vi "Chanel Names.vi"(7 "Write?":bool, 8 "error in":errorcluster, 10 "Channel Names":T1={"A-1,  1"="Main", "A-3,  2"="Main", "A-4, 3"="Recirculation", "A-5, 4"="Scrubber", "ABCD-7, 5"="Oxygen", "D-8, 6"="Vent", "B-1,  7"="Boost A", "B-3, 8"="Boost A", "B-4,  9"="Recirculation", "B-5, 10"="Scrubber", "B-8, 11"="Vent", "C-1, 12"="Boost B", "C-3, 13"="Boost B", "C-4, 14"="Recirculation", "C-5,  15"="Scrubber", "C-8, 16"="Vent", "D-1, 17"="+24V", "D-3, 18"="Main", "D-4,  19"="Boost A", "D-5,  20"="Boost B", "D-8,  21"="Vent"}, 11 "CfgFileIn":T2) -> (0 "error out":errorcluster, 2 "Channel Names Out":T1={"A-1,  1"="Main", "A-3,  2"="Main", "A-4, 3"="Recirculation", "A-5, 4"="Scrubber", "ABCD-7, 5"="Oxygen", "D-8, 6"="Vent", "B-1,  7"="Boost A", "B-3, 8"="Boost A", "B-4,  9"="Recirculation", "B-5, 10"="Scrubber", "B-8, 11"="Vent", "C-1, 12"="Boost B", "C-3, 13"="Boost B", "C-4, 14"="Recirculation", "C-5,  15"="Scrubber", "C-8, 16"="Vent", "D-1, 17"="+24V", "D-3, 18"="Main", "D-4,  19"="Boost A", "D-5,  20"="Boost B", "D-8,  21"="Vent"}, 3 "CfgFileOut":T2)   [LabVIEW 2012]
uses:
  <vilib>/Utility/config.llb/Config Data RefNum.ctl
  Type Defs/Named Final Output name list ordered.ctl
  <vilib>/Utility/config.llb/Write Key (String).vi
  <vilib>/Utility/config.llb/Read Key (String).vi
  <vilib>/Utility/config.llb/NI_LVConfig.lvlib
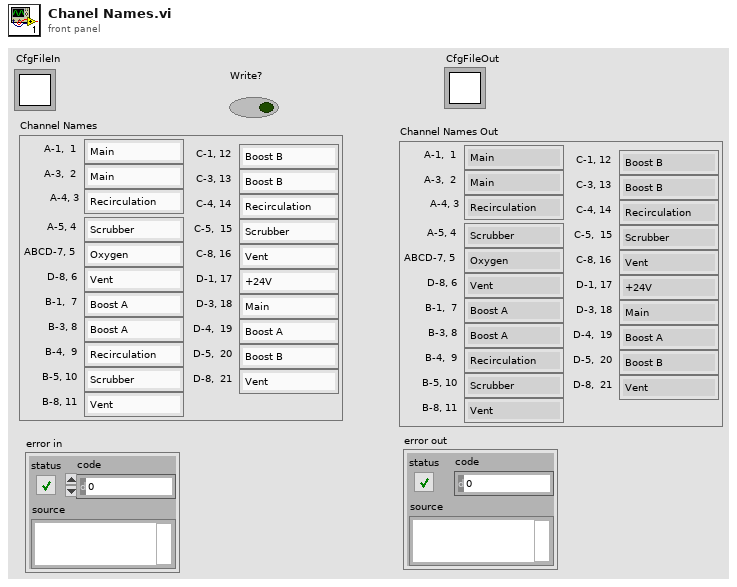
[diagram p1: front panel]
types:
  T1 = typedef "Named Final Output name list ordered.ctl" = cluster{"A-1,  1":string, "A-3,  2":string, "A-4, 3":string, "A-5, 4":string, "ABCD-7, 5":string, "D-8, 6":string, "B-1,  7":string, "B-3, 8":string, "B-4,  9":string, "B-5, 10":string, "B-8, 11":string, "C-1, 12":string, "C-3, 13":string, "C-4, 14":string, "C-5,  15":string, "C-8, 16":string, "D-1, 17":string, "D-3, 18":string, "D-4,  19":string, "D-5,  20":string, "D-8,  21":string}
  T2 = typedef "NI_LVConfig.lvlib/Config Data RefNum.ctl" = refnum<k1>
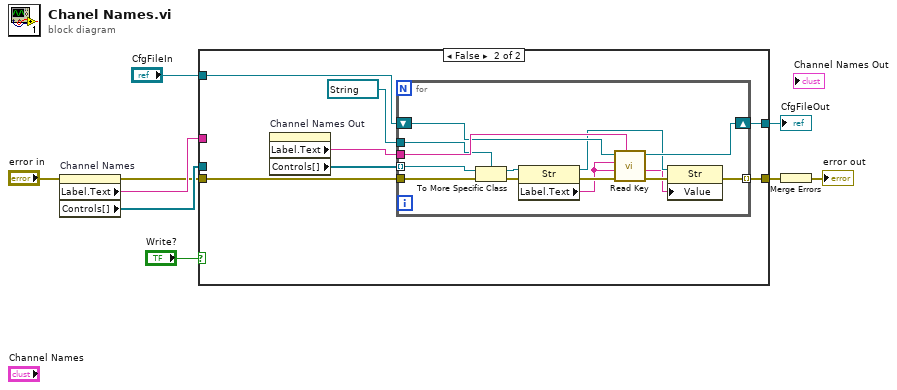
[diagram p0: block diagram]
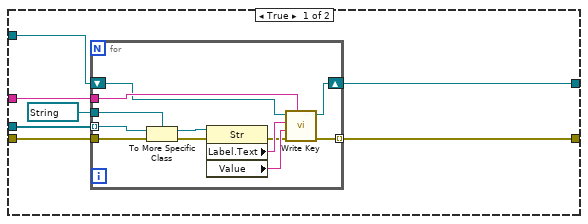
[diagram p2: hidden frame]
diagram:
  n1 = property on="Channel Names" class="Clust (strict)"(error in="error in") -> (error out=w4:errorcluster, "Label.Text"=w8:string, "Controls[]"=w9:refnum<vi>[])  [unwired: 1 in, 1 out]
  n2 = case shown="False" "Write?" {
    tunnel: w9 -> [w16 _]
    tunnel: w8 -> [w15 _]
    tunnel: "CfgFileIn" -> [w13 w34]
    tunnel: [w12 w33] -> w6
    tunnel: w4 -> [w11 w32]
    tunnel: [w10 w31] -> w3
    frame True {
      n3 = for {
        tunnel: w16 -> [w27] mode=indexing
        tunnel: w15 -> [w28]
        tunnel: refnum<vi> refnum ("Str Refnum") -> [w26]
        shift-right: [w20] -> w12
        shift-left: w13 -> [w23]
        tunnel: w11 -> [w19]
        tunnel: [w17] -> w10 mode=indexing
        n4 = To More Specific Class(target class=w26, reference=w27, error in=w19) -> (specific class reference=w25:refnum<vi>, error out=w24:errorcluster)
        n5 = property class="Str"(reference=w25, error in=w24) -> (error out=w18:errorcluster, "Label.Text"=w22:string, "Value"=w21:string)  [unwired: 1 out]
        n6 = call-poly <vilib>:"Write Key.vi"("section"=w28, "error in (no error)"=w18, "value"=w21, "key"=w22, "refnum"=w23) -> ("error out"=w17:errorcluster, "refnum out"=w20:T2)  [unwired: 4 in, 1 out]
      }
    }
    frame False {
      n7 = property on="Channel Names Out" class="Clust (strict)"() -> ("Label.Text"=w30:string, "Controls[]"=w29:refnum<vi>[])  [unwired: 2 in, 2 out]
      n8 = for {
        tunnel: w29 -> [w40] mode=indexing
        tunnel: w30 -> [w49]
        tunnel: refnum<vi> refnum ("Str Refnum") -> [w48]
        shift-right: [w44] -> w33
        shift-left: w34 -> [w45]
        tunnel: w32 -> [w43]
        tunnel: [w37] -> w31 mode=indexing
        n9 = To More Specific Class(target class=w48, reference=w40, error in=w43) -> (specific class reference=w47:refnum<vi>, error out=w46:errorcluster)
        n10 = property class="Str"(reference=w47, error in=w46) -> (reference out=w39:refnum<vi>, error out=w42:errorcluster, "Label.Text"=w41:string)
        n11 = call-poly <vilib>:"Read Key.vi"("section"=w49, "error in (no error)"=w42, "default value"=w41, "key"=w41, "refnum"=w45) -> ("error out"=w38:errorcluster, "value"=w36:string, "refnum out"=w44:T2)  [unwired: 3 in, 1 out]
        n12 = property class="Str"(reference=w39, error in=w38, "Value"=w36) -> (error out=w37:errorcluster)  [unwired: 1 out]
      }
    }
  }
  "CfgFileOut" <- w6
  n13 = Merge Errors(w3) -> (→"error out":errorcluster)
